vi "Auto Lifter.vi"(11 "MechanismMetrics in":T1) -> (3 "MechanismMetrics in 2":T1)   [LabVIEW 2014]
uses:
  MechanismMetrics.ctl
  Lifter States.ctl
  Auto Lifter States.ctl
  <vilib>/Rock Robotics/WPI/Solenoid/WPI_SolenoidValue.ctl
  Lifter Hights.vi
  <vilib>/Rock Robotics/WPI/Solenoid/WPI_SolenoidSetEnum.vi
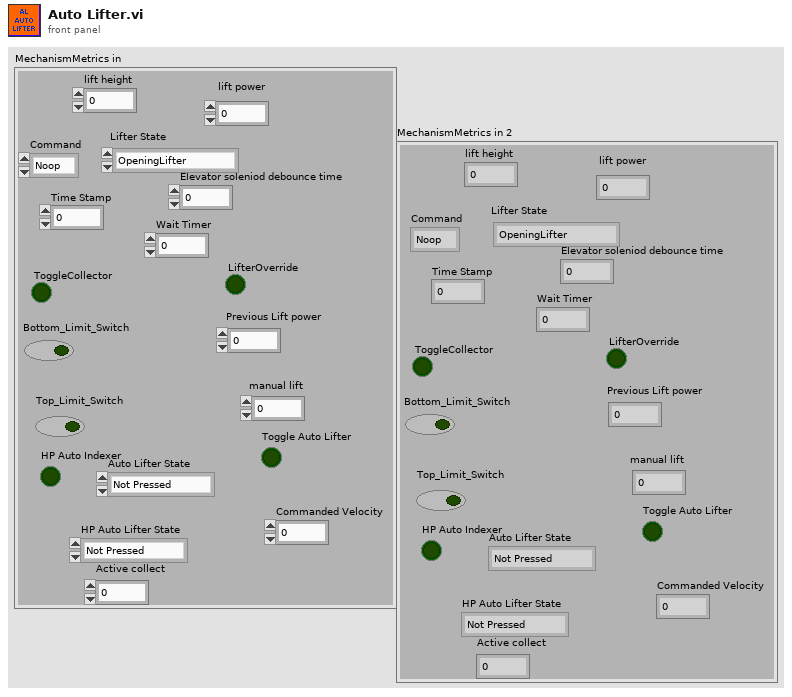
[diagram p1: front panel]
types:
  T1 = typedef "MechanismMetrics.ctl" = cluster{"lift height":dbl, "Command":enum16{"Noop", "Flagged"}, "Time Stamp":u32, "ToggleCollector":bool, "Bottom_Limit_Switch ":bool, "Top_Limit_Switch":bool, "lift power":dbl, "Elevator soleniod debounce time   ":dbl, "LifterOverride":bool, "Previous Lift power":dbl, "manual lift":dbl, "Lifter State":T2, "Auto Lifter State":T3, "Toggle Auto Lifter":bool, "Wait Timer":dbl, "HP Auto Indexer":bool, "HP Auto Lifter State":T3, "Commanded Velocity":dbl, "\nActive collect":dbl}
  T2 = typedef "Lifter States.ctl" = enum16{"OpeningLifter", "LifterOpen", "ClosingLifter", "LifterClosed"}
  T3 = typedef "Auto Lifter States.ctl" = enum16{"Not Pressed", "THE_END", "WAIT_FOR_RELEASE", "Press Detected", "To Release Stacked1", "To Collect", "Open Lifter", "WAIT", "Close", "To Stack1"}
  T4 = typedef "WPI_SolenoidValue.ctl" = enum16{"Off", "On", "Forward", "Reverse"}
  T5 = typedef "WPI_SolenoidDevRef.ctl" = cluster{"DevStatus":errorcluster, "Pneumatics Control Module":u8, "Forward Solenoid Channel":T6, "Reverse Solenoid Channel":T6}
  T6 = typedef "WPI_SolenoidChannel.ctl" = enum8{"Solenoid 0", "Solenoid 1", "Solenoid 2", "Solenoid 3", "Solenoid 4", "Solenoid 5", "Solenoid 6", "Solenoid 7", "Invalid"}
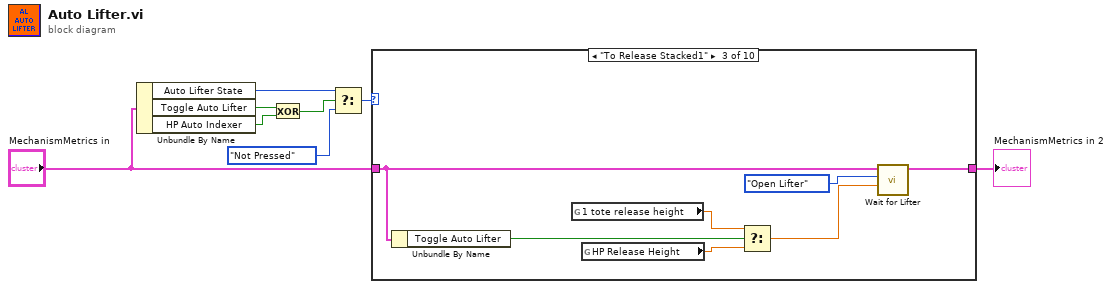
[diagram p0: block diagram]
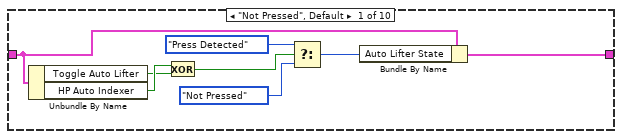
[diagram p2: hidden frame]
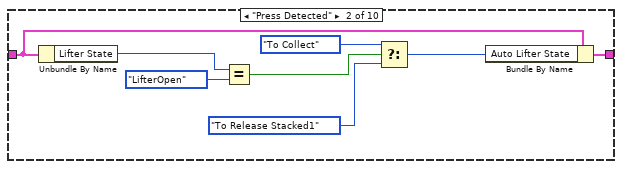
[diagram p3: hidden frame]
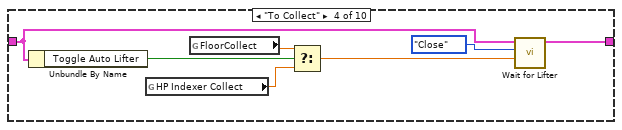
[diagram p4: hidden frame]
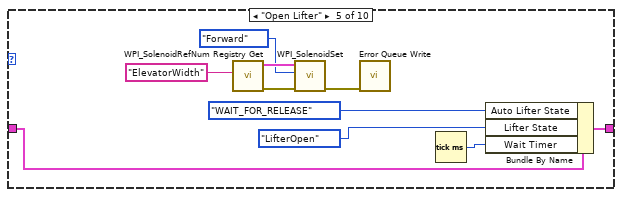
[diagram p5: hidden frame]
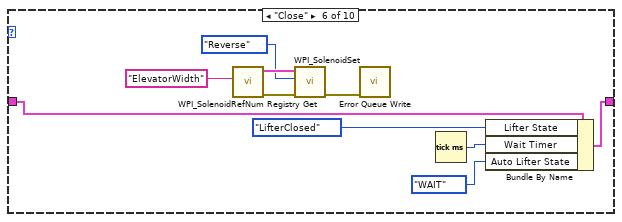
[diagram p6: hidden frame]
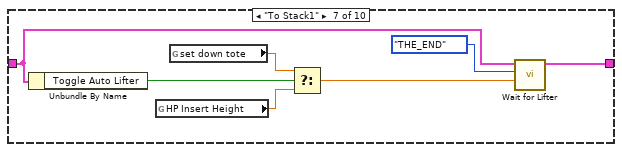
[diagram p7: hidden frame]
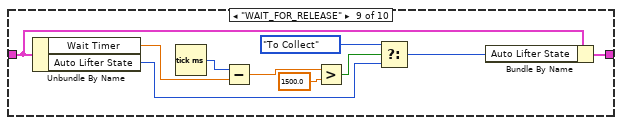
[diagram p9: hidden frame]
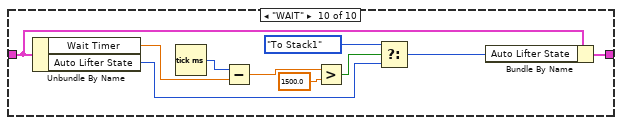
[diagram p10: hidden frame]
diagram:
  n1 = Unbundle By Name("MechanismMetrics in") -> ("Auto Lifter State"=w6:T3, "Toggle Auto Lifter"=w3:bool, "HP Auto Indexer"=w1:bool)
  n2 = Exclusive Or(1:w1, 2:w3) -> (0:w2:bool)
  n3 = Select(t=w6, s=w2, f=Auto_Lifter_States."Not Pressed") -> (s? t:f=w4:T3)
  n4 = case shown="\"To Release Stacked1\"" w4 {
    tunnel: "MechanismMetrics in" -> [w14 w19 w26 w33 w41 w52 w61 w66 w76 w81]
    tunnel: [w12 w17 w30 w37 w40 w53 w64 w66 w75 w77] -> w8
    frame "Not Pressed", Default {
      n5 = Unbundle By Name(w14) -> ("Toggle Auto Lifter"=w10:bool, "HP Auto Indexer"=w11:bool)
      n6 = Exclusive Or(1:w10, 2:w11) -> (0:w9:bool)
      n7 = Select(t=Auto_Lifter_States."Press Detected", s=w9, f=Auto_Lifter_States."Not Pressed") -> (s? t:f=w13:T3)
      n8 = Bundle By Name(cluster=w14, "Auto Lifter State"=w13) -> (w12:T1)
    }
    frame "Press Detected" {
      n9 = Unbundle By Name(w19) -> ("Lifter State"=w24:T2)
      n10 = Equal?(x=w24, y=Lifter_States."LifterOpen" ("Lifter States")) -> (x = y?=w22:bool)
      n11 = Select(t=Auto_Lifter_States."To Collect", s=w22, f=Auto_Lifter_States."To Release Stacked1") -> (s? t:f=w18:T3)
      n12 = Bundle By Name(cluster=w19, "Auto Lifter State"=w18) -> (w17:T1)
    }
    frame "To Release Stacked1" {
      n13 = Unbundle By Name(w26) -> ("Toggle Auto Lifter"=w25:bool)
      n14 = global read "Lifter Hights.vi" "1 tote release height"() -> (w29:dbl)
      n15 = global read "Lifter Hights.vi" "HP Release Height"() -> (w27:dbl)
      n16 = Select(t=w29, s=w25, f=w27) -> (s? t:f=w28:dbl)
      n17 = call "Wait for Lifter.vi"("1 tote high"=w28, "Auto Lifter States"=Auto_Lifter_States."Open Lifter", "MechanismMetrics in in"=w26) -> ("MechanismMetrics out"=w30:T1)  [unwired: 8 in]
    }
    frame "To Collect" {
      n18 = Unbundle By Name(w33) -> ("Toggle Auto Lifter"=w32:bool)
      n19 = global read "Lifter Hights.vi" "HP Indexer Collect"() -> (w34:dbl)
      n20 = global read "Lifter Hights.vi" "FloorCollect"() -> (w36:dbl)
      n21 = Select(t=w36, s=w32, f=w34) -> (s? t:f=w35:dbl)
      n22 = call "Wait for Lifter.vi"("1 tote high"=w35, "Auto Lifter States"=Auto_Lifter_States."Close", "MechanismMetrics in in"=w33) -> ("MechanismMetrics out"=w37:T1)  [unwired: 8 in]
    }
    frame "Open Lifter" {
      n23 = call <vilib>:"WPI_SolenoidRefNum Registry Get.vi"("refnum name"="ElevatorWidth") -> ("error out"=w48:errorcluster, "SolenoidDevRef"=w47:T5)  [unwired: 9 in]
      n24 = call-poly <vilib>:"WPI_SolenoidSet.vi"("error in (no error)"=w48, "Value"=WPI_SolenoidValue."Forward", "SolenoidDevRef"=w47) -> ("error out"=w45:errorcluster)  [unwired: 7 in, 1 out]
      n25 = call "Error Queue Write.vi"("error in (no error)"=w45) -> ()  [unwired: 11 in]
      n26 = Tick Count (ms)() -> (millisecond timer value=w43:u32)
      n27 = Bundle By Name(cluster=w41, "Auto Lifter State"=Auto_Lifter_States."WAIT_FOR_RELEASE" ("f"), "Lifter State"=Lifter_States."LifterOpen" ("Lifter States"), "Wait Timer"=w43) -> (w40:T1)
    }
    frame "Close" {
      n28 = call <vilib>:"WPI_SolenoidRefNum Registry Get.vi"("refnum name"="ElevatorWidth") -> ("error out"=w56:errorcluster, "SolenoidDevRef"=w57:T5)  [unwired: 9 in]
      n29 = call-poly <vilib>:"WPI_SolenoidSet.vi"("error in (no error)"=w56, "Value"=WPI_SolenoidValue."Reverse", "SolenoidDevRef"=w57) -> ("error out"=w58:errorcluster)  [unwired: 7 in, 1 out]
      n30 = call "Error Queue Write.vi"("error in (no error)"=w58) -> ()  [unwired: 11 in]
      n31 = Tick Count (ms)() -> (millisecond timer value=w50:u32)
      n32 = Bundle By Name(cluster=w52, "Lifter State"=Lifter_States."LifterClosed" ("Lifter States"), "Wait Timer"=w50, "Auto Lifter State"=Auto_Lifter_States."WAIT" ("f")) -> (w53:T1)
    }
    frame "To Stack1" {
      n33 = Unbundle By Name(w61) -> ("Toggle Auto Lifter"=w59:bool)
      n34 = global read "Lifter Hights.vi" "HP Insert Height"() -> (w62:dbl)
      n35 = global read "Lifter Hights.vi" "set down tote"() -> (w63:dbl)
      n36 = Select(t=w63, s=w59, f=w62) -> (s? t:f=w60:dbl)
      n37 = call "Wait for Lifter.vi"("1 tote high"=w60, "Auto Lifter States"=Auto_Lifter_States."THE_END", "MechanismMetrics in in"=w61) -> ("MechanismMetrics out"=w64:T1)  [unwired: 8 in]
    }
    frame "THE_END" {
    }
    frame "WAIT_FOR_RELEASE" {
      n38 = Unbundle By Name(w76) -> ("Wait Timer"=w68:dbl, "Auto Lifter State"=w71:T3)
      n39 = Tick Count (ms)() -> (millisecond timer value=w69:u32)
      n40 = Subtract(x=w69, y=w68) -> (x-y=w67:dbl)
      n41 = Greater?(x=w67, y=1500.0) -> (0:w73:bool)
      n42 = Select(t=Auto_Lifter_States."To Collect", s=w73, f=w71) -> (s? t:f=w72:T3)
      n43 = Bundle By Name(cluster=w76, "Auto Lifter State"=w72) -> (w75:T1)
    }
    frame "WAIT" {
      n44 = Unbundle By Name(w81) -> ("Wait Timer"=w79:dbl, "Auto Lifter State"=w83:T3)
      n45 = Tick Count (ms)() -> (millisecond timer value=w80:u32)
      n46 = Subtract(x=w80, y=w79) -> (x-y=w78:dbl)
      n47 = Greater?(x=w78, y=1500.0) -> (0:w85:bool)
      n48 = Select(t=Auto_Lifter_States."To Stack1", s=w85, f=w83) -> (s? t:f=w84:T3)
      n49 = Bundle By Name(cluster=w81, "Auto Lifter State"=w84) -> (w77:T1)
    }
  }
  "MechanismMetrics in 2" <- w8
